vi "Read RLNA URL.vi"(8 "error in (no error)":errorcluster, 11 "Test LNA in":refnum<class "TestLNA.lvclass">) -> (0 "error out":errorcluster, 2 "RLNA URL":string, 3 "Test LNA out":refnum<class "TestLNA.lvclass">)   [LabVIEW 2015, in "TestLNA.lvlib" / "TestLNA.lvclass"]
uses:
  TestLNA.lvclass
  TestLNA.lvclass/TestLNA.ctl
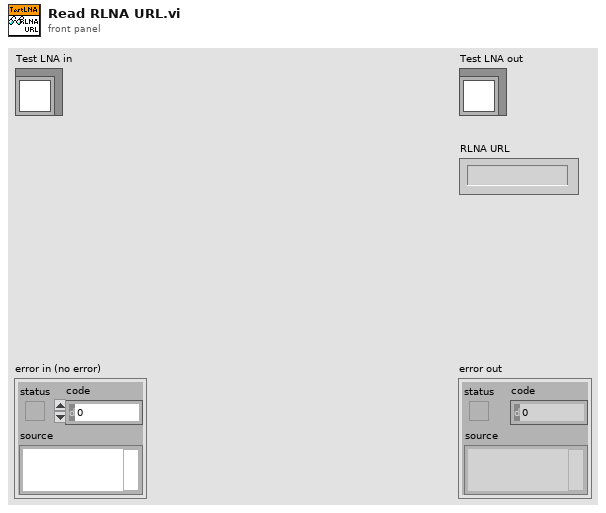
[diagram p1: front panel]
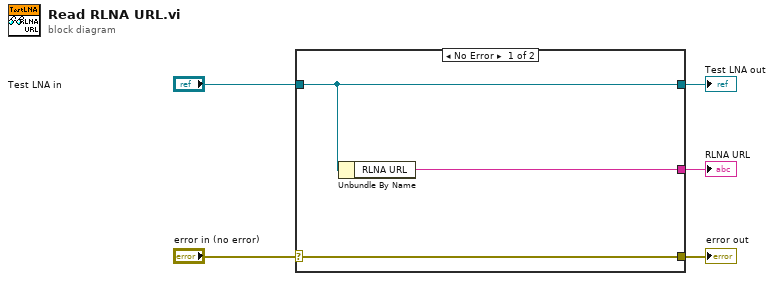
[diagram p0: block diagram]
diagram:
  n1 = case shown="No Error" "error in (no error)" {
    selector: "error in (no error)" -> [w8 w9]
    tunnel: [w8 w9] -> w4
    tunnel: [w7 w10] -> w2
    tunnel: "Test LNA in" -> [w7 w10]
    tunnel: [w6 _] -> w1
    frame No Error {
      n2 = Unbundle By Name(w7) -> ("RLNA URL"=w6:string)
    }
    frame Error {
    }
  }
  "error out" <- w4
  "Test LNA out" <- w2
  "RLNA URL" <- w1
